vi "WSVCAP SHL Host TL SPI Write_Read - Multiple DUTs - Common Data.vi"(0 "Data Out":string, 11 "error in":errorcluster, 13 "DUT Mask (All)":bool[](array[boolean])=[TRUE, TRUE, TRUE, TRUE, TRUE, TRUE, TRUE, TRUE, TRUE, TRUE, TRUE, TRUE, TRUE, TRUE, TRUE, TRUE]) -> (4 "SPI Data In":string[](array[string]), 15 "error out":errorcluster)   [LabVIEW 2012]
panel:
  out "SPI Data In [U8]":u8[][](array[numeric]) format="%02x"
  out "Socket Mask":u16=1 format="%02x"
  out "SPI Data Out [U8]":u8[][](array[numeric]) format="%02x"
  # "DUT 01"
  # "DUT 02"
  # "DUT 03"
  # "DUT 04"
  # "DUT 05"
  # "DUT 06"
  # "DUT 07"
  # "DUT 08"
  # "DUT 09"
  # "DUT 10"
  # "DUT 11"
  # "DUT 12"
  # "DUT 13"
  # "DUT 14"
  # "DUT 15"
  # "DUT 16"
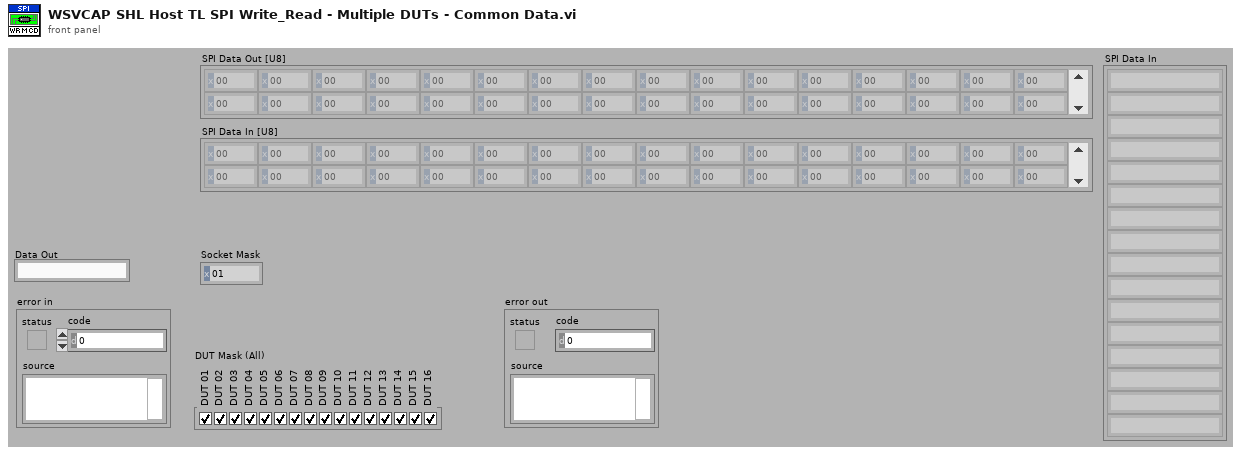
[diagram p1: front panel]
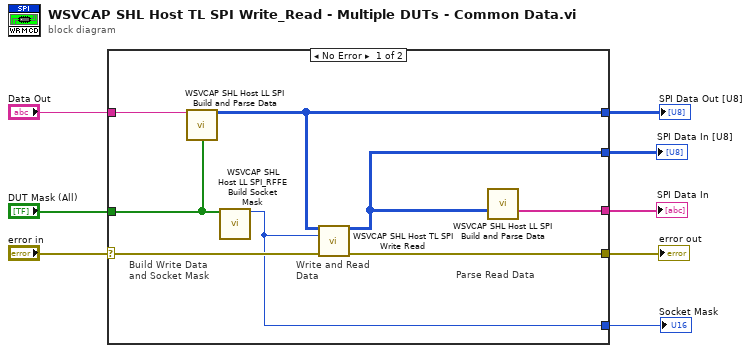
[diagram p0: block diagram]
diagram:
  n1 = case shown="No Error" "error in" {
    selector: "error in" -> [w15 _]
    tunnel: [w16 _] -> w8
    tunnel: "Data Out" -> [w14 _]
    tunnel: [w12 _] -> w5
    tunnel: [w11 _] -> w4
    tunnel: "DUT Mask (All)" -> [w13 _]
    tunnel: [w10 _] -> w2
    tunnel: [w9 _] -> w1
    frame No Error {
      # "Parse Read Data"
      # "Write and Read\nData"
      # "Build Write Data and Socket Mask"
      n2 = call "WSVCAP SHL Host LL SPI Build and Parse Data.vi"("Data Out"=w14, "DUT Mask (All)"=w13) -> ("SPI Data Out [U8]"=w12:u8[][])  [unwired: 10 in, 3 out]
      n3 = call "WSVCAP SHL Host LL SPI_RFFE Build Socket Mask.vi"("DUT Mask"=w13) -> ("Socket Mask [U16]"=w11:u16)  [unwired: 13 in, 1 out]
      n4 = call "WSVCAP SHL Host TL SPI Write Read.vi"("SPI Data Out"=w12, "Socket Mask"=w11, "error in"=w15) -> ("Read Data Out"=w10:u8[][], "error out"=w16:errorcluster)  [unwired: 11 in]
      n5 = call "WSVCAP SHL Host LL SPI Build and Parse Data.vi"("SPI Data In [U8]"=w10) -> ("SPI Data In"=w9:string[])  [unwired: 11 in, 3 out]
    }
    frame Error {
    }
  }
  "error out" <- w8
  "SPI Data Out [U8]" <- w5
  "Socket Mask" <- w4
  "SPI Data In" <- w1
  "SPI Data In [U8]" <- w2
